vi "Write Serial data.vi"(8 "error in":errorcluster, 10 "PAS Data In":refnum<class "PAS Data.lvclass">=refnum, 11 "File Obs in":refnum<class "PAS File Obs.lvclass">) -> (0 "error out":errorcluster, 2 "PAS Data Out":refnum<class "PAS Data.lvclass">, 3 "File Obs Out":refnum<class "PAS File Obs.lvclass">)   [LabVIEW 2014, in "PAS File Obs.lvclass"]
uses:
  PAS File Obs.lvclass
  Main/Controls/pas_data_enum.ctl
  Devices/TE Cooler/Data/TECData.lvclass
  Devices/Alicat/Data/MC/AlicatMCData.lvclass
  Main/Controls/Cell Data.ctl
  Data/Main/PAS Data.lvclass
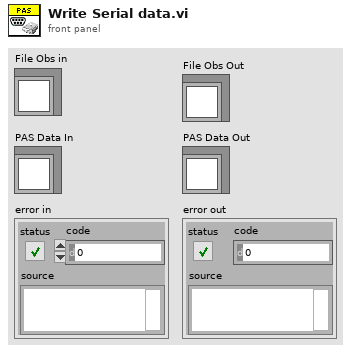
[diagram p1: front panel]
types:
  T1 = enum16{"big-endian, network order", "native, host order", "little-endian"}
  T2 = cluster{"P":sgl, "T":sgl, "Q":sgl, "Q0":sgl, "Qsp":sgl}
  T3 = typedef "Cell Data.ctl" = u8
  T4 = typedef "pas_data_enum.ctl" = enum8{"Time", "Ttec", "tecPow", "Spk Position", "Spk Amplification", "Vspan", "Modulation", "Vspk", "Filter", "DC State", "Notes", "O3 Flag", "Raw Flags"}
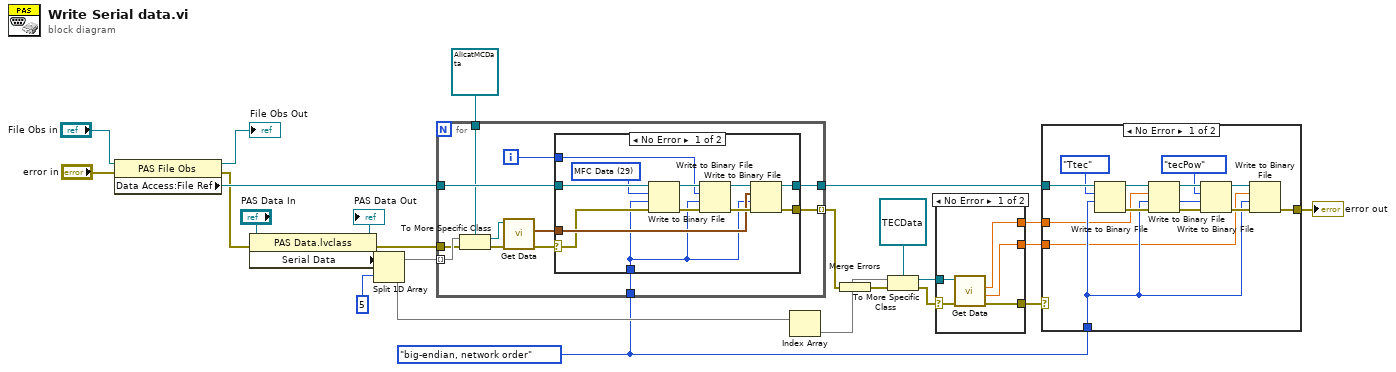
[diagram p0: block diagram]
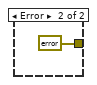
[diagram p3: hidden frame]
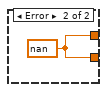
[diagram p4: hidden frame]
diagram:
  w8 = T1."big-endian, network order" ("byte order (0:big-endian, network order)")
  n1 = property class="PAS File Obs"(reference="File Obs in", error in="error in") -> (reference out=→"File Obs Out":refnum<class "PAS File Obs.lvclass">, error out=w3:errorcluster, "Data Access:File Ref"=w10:refnum<file>)
  n2 = property class="PAS Data.lvclass"(reference="PAS Data In", error in=w3) -> (reference out=→"PAS Data Out":refnum<class "PAS Data.lvclass">, error out=w9:errorcluster, "Serial Data"=w15)
  n3 = Split 1D Array(array=w15, index=5) -> (first subarray=w11:void[], second subarray=w23:void[])
  n4 = for {
    tunnel: w11 -> [w33] mode=indexing
    tunnel: w10 -> [w32]
    tunnel: [w31] -> w7
    tunnel: w9 -> [w30]
    tunnel: w8 -> [w29]
    tunnel: [w27] -> w6 mode=indexing
    tunnel: refnum<class "AlicatMCData.lvclass"> refnum ("Alicat.lvlib:AlicatMCData.lvclass") -> [w26]
    i -> [w28]
    n5 = To More Specific Class(target class=w26, reference=w33, error in=w30) -> (specific class reference=w37:refnum<class "AlicatMCData.lvclass">, error out=w36:errorcluster)
    n6 = call "Get Data.vi"("error in"=w36, "AlicatMData in"=w37) -> ("error out"=w34:errorcluster, "SystemData"=w35:T2)  [unwired: 7 in, 1 out]
    n7 = case shown="No Error" w34 {
      selector: w34 -> [w39 w50]
      tunnel: w32 -> [w49 w51]
      tunnel: w35 -> [w44 _]
      tunnel: [w43 w50] -> w27
      tunnel: [w41 w51] -> w31
      tunnel: w29 -> [w38 _]
      tunnel: w28 -> [w40 _]
      frame No Error {
        w42 = T3 29 items=["TEC SP"=23, "TEC Enable"=24, "MFC Data"=29, "Cell TEC T (T1)"=30, "Tmain"=31, "Tv"=32, "RHv"=33, "lasRMS"=34, "dPhi"=35, "Tau"=36, "Cell Q"=37, "f0"=38, "Integrated Area"=39, "Max Amplitude"=40, "Noise Limit"=41, "Lower Noise Bound"=42, "Upper Noise Bound"=43, "Absorption"=44, "fit params"=45, "covariance"=46] ("cellNumData")
        n8 = Write to Binary File(file (use dialog)=w49, data=w42, error in=w39, 9:w38) -> (refnum out=w48:refnum<file>, error out=w47:errorcluster)  [unwired: 2 in, 1 out]
        n9 = Write to Binary File(file (use dialog)=w48, data=w40, error in=w47, 9:w38) -> (refnum out=w46:refnum<file>, error out=w45:errorcluster)  [unwired: 2 in, 1 out]
        n10 = Write to Binary File(file (use dialog)=w46, data=w44, error in=w45, 9:w38) -> (refnum out=w41:refnum<file>, error out=w43:errorcluster)  [unwired: 2 in, 1 out]
      }
      frame Error {
      }
    }
  }
  n11 = Index Array(array=w23) -> (element=w14)  [unwired: 1 in]
  n12 = Merge Errors(w6) -> (w5:errorcluster)
  n13 = To More Specific Class(target class=refnum<class "TECData.lvclass"> refnum ("TE Cooler.lvlib:TECData.lvclass"), reference=w14, error in=w5) -> (specific class reference=w19:refnum<class "TECData.lvclass">, error out=w21:errorcluster)
  n14 = case shown="No Error" w21 {
    selector: w21 -> [w53 _]
    tunnel: w19 -> [w56 _]
    tunnel: [w55 w57] -> w20
    tunnel: [w54 _] -> w25
    tunnel: [w52 w57] -> w24
    frame No Error {
      n15 = call "Get Data.vi"("error in (no error)"=w53, "TECData in"=w56) -> ("error out"=w54:errorcluster, "Power"=w52:sgl, "T"=w55:sgl)  [unwired: 6 in, 1 out]
    }
    frame Error {
      w57 = sgl nan ("T")
    }
  }
  n16 = case shown="No Error" w25 {
    tunnel: [w68 errorcluster {"status"=FALSE, "code"=0, "source"=""} ("error out")] -> w17
    tunnel: w20 -> [w59 _]
    tunnel: w8 -> [w62 _]
    tunnel: w24 -> [w58 _]
    tunnel: w7 -> [w63 _]
    frame No Error {
      n17 = Write to Binary File(file (use dialog)=w63, data=pas_data_enum."Ttec" ("Enum"), 9:w62) -> (refnum out=w67:refnum<file>, error out=w64:errorcluster)  [unwired: 3 in, 1 out]
      n18 = Write to Binary File(file (use dialog)=w67, data=w59, error in=w64, 9:w62) -> (refnum out=w66:refnum<file>, error out=w65:errorcluster)  [unwired: 2 in, 1 out]
      n19 = Write to Binary File(file (use dialog)=w66, data=pas_data_enum."tecPow" ("Enum"), error in=w65, 9:w62) -> (refnum out=w69:refnum<file>, error out=w70:errorcluster)  [unwired: 2 in, 1 out]
      n20 = Write to Binary File(file (use dialog)=w69, data=w58, error in=w70, 9:w62) -> (error out=w68:errorcluster)  [unwired: 2 in, 2 out]
    }
    frame Error {
    }
  }
  "error out" <- w17
